vi "PreLoop.vi"(8 "error in":errorcluster, 11 "VI Ref":refnum<vi>) -> (0 "error out":errorcluster, 3 "Event Registration Refnum":refnum<event-registration>)   [LabVIEW 2018, in "S4.lvclass"]
uses:
  S4.lvclass
  Queue/Queue.ctl
  Controller/GUI.lvclass
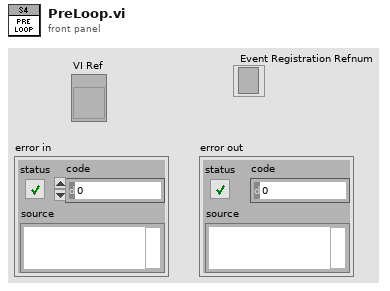
[diagram p1: front panel]
types:
  T1 = typedef "S4.lvclass/Queue.ctl" = enum16{"Create", "Get", "Destroy"}
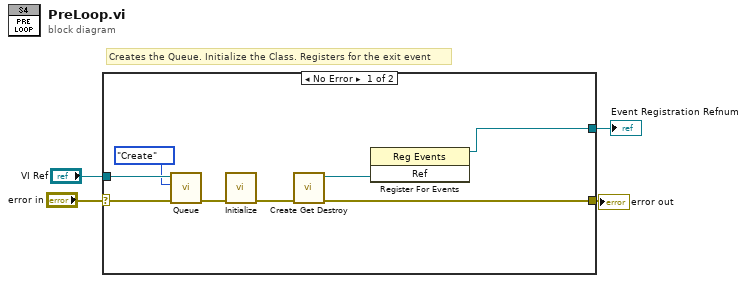
[diagram p0: block diagram]
diagram:
  # "Creates the Queue. Initialize the Class. Registers for the exit event"
  n1 = case shown="No Error" "error in" {
    selector: "error in" -> [w12 _]
    tunnel: [w7 _] -> w4
    tunnel: "VI Ref" -> [w11 _]
    tunnel: [w5 _] -> w1
    frame No Error {
      n2 = call "Queue.vi"("error in"=w12, "State(Get)"=Queue."Create" ("State"), "VI Ref"=w11) -> ("error out"=w9:errorcluster)  [unwired: 7 in, 1 out]
      n3 = call "Initialize.vi"("error in"=w9) -> ("error out"=w8:errorcluster)  [unwired: 10 in]
      n4 = call "Create Get Destroy.vi"("error In"=w8) -> ("Error Out"=w7:errorcluster, "Ref"=w6:refnum<user-event>)  [unwired: 9 in]
      n5 = register-events(w6) -> (reference out=w5:refnum<event-registration>)  [unwired: 2 in, 1 out]
    }
    frame Error {
    }
  }
  "error out" <- w4
  "Event Registration Refnum" <- w1
